vi "Version 1_Save Register Values.vi"(7 "Address (A)":string="A", 8 "error in":errorcluster, 10 "file path":path, 11 "VISA Session In":refnum<visa-resource-name>="Alicat") -> (0 "error out":errorcluster, 3 "VISA Session Out":refnum<visa-resource-name>)   [LabVIEW 2015]
uses:
  <vilib>/Utility/file.llb/Write To Spreadsheet File (string).vi
panel:
  # "Code left un-changed.\nFor use of the newer code, \nuse the \"Log Current Register\nValues.vi\""
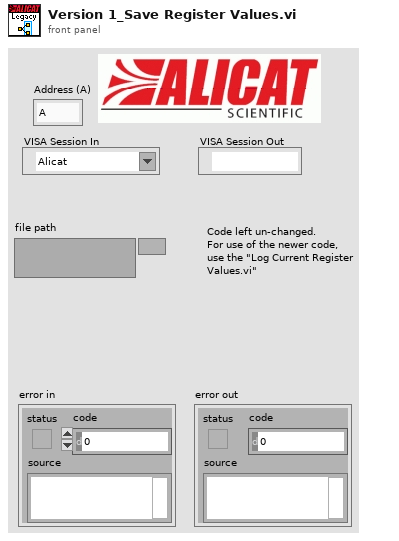
[diagram p1: front panel]
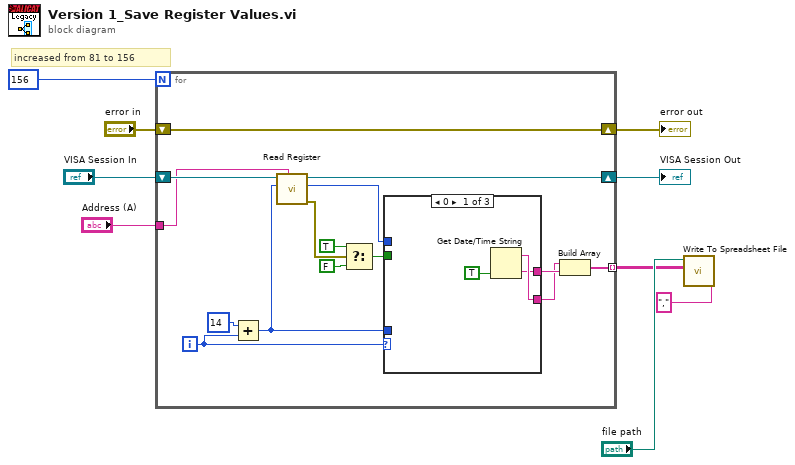
[diagram p0: block diagram]
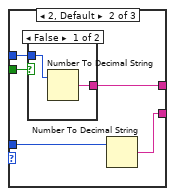
[diagram p2: hidden frame]
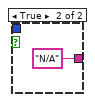
[diagram p3: hidden frame]
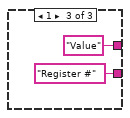
[diagram p4: hidden frame]
diagram:
  # "increased from 81 to 156"
  n1 = for {
    N: 156 -> [_]
    tunnel: "Address (A)" -> [w23]
    shift-right: [w22] -> w6
    shift-left: "VISA Session In" -> [w24]
    shift-right: [w20] -> w5
    shift-left: "error in" -> [w20]
    tunnel: [w10] -> w1 mode=indexing
    i -> [w13]
    n2 = Add(x=14, y=w13) -> (x+y=w19:i32)
    n3 = call "Read Register.vi"("Unit ID (A)"=w23, "Register address"=w19, "VISA Session In"=w24) -> ("error out"=w18:errorcluster, "Register Value (I32)"=w15:i32, "VISA Session Out"=w22:refnum<visa-resource-name>)  [unwired: 6 in]
    n4 = Select(t=TRUE, s=w18, f=FALSE) -> (s? t:f=w14:bool)
    n5 = case shown="0" w13 {
      tunnel: w19 -> [_ w32 _]
      tunnel: w15 -> [_ w31 _]
      tunnel: w14 -> [_ w30 _]
      tunnel: [w26 w29 "Value"] -> w12
      tunnel: [w27 w28 "Register #"] -> w11
      frame 0 {
        n6 = Get Date/Time String(want seconds? (F)=TRUE) -> (date string=w27:string, time string=w26:string)  [unwired: 2 in]
      }
      frame 2, Default {
        n7 = case shown="False" w30 {
          tunnel: [w34 "N/A"] -> w29
          tunnel: w31 -> [w33 _]
          frame False {
            n8 = Number To Decimal String(number=w33) -> (decimal integer string=w34:string)  [unwired: 1 in]
          }
          frame True {
          }
        }
        n9 = Number To Decimal String(number=w32) -> (decimal integer string=w28:string)  [unwired: 1 in]
      }
      frame 1 {
      }
    }
    n10 = Build Array(w11, w12) -> (w10:string[])
  }
  "error out" <- w5
  "VISA Session Out" <- w6
  n11 = call-poly <vilib>:"Write To Spreadsheet File.vi"("delimiter (\\t)"="," ("delimiter (\\t)"), "2D data"=w1, "file path (dialog if empty)"="file path") -> ()  [unwired: 5 in, 1 out]
